vi "Teleop.vi"(10 "Match Info":T1={"Autonomous Elapsed Seconds"=0.0, "TeleOp Elapsed Seconds"=0.0, "Disabled Elapsed Seconds"=0.0, "Visited Autonomous"=FALSE, "Visited TeleOp"=FALSE, "Visited Disabled"=FALSE, "Autonomous Settings"={"Autonomous Style"=enum."Independent", "VI Refnum"=refnum}}, 11 "Call Context":T2) -> ()   [LabVIEW 2014]
doc: "This VI is called for each TeleOp packet received from the DS where the robot is not disabled. It is often used to read from the joysticks and update I/O or to update setpoints for timed control loops. It should complete and return within 20 milliseconds or it may miss DS packets."
uses:
  <vilib>/Rock Robotics/WPI/DriverStation/WPI_DriverStationDerivedRobotMode.ctl
  <vilib>/Rock Robotics/WPI/DriverStation/WPI_DriverStationMatch Info.ctl
  <vilib>/Rock Robotics/WPI/Solenoid/WPI_SolenoidValue.ctl
  <vilib>/Rock Robotics/WPI/RobotDrive/WPI_RobotDriveGetSetRefNum.vi
  <vilib>/Rock Robotics/WPI/Joystick/WPI_JoystickGetSetRefNum.vi
  Robot Global Data.vi
  <vilib>/Rock Robotics/WPI/Solenoid/WPI_SolenoidSetEnum.vi
  <vilib>/Rock Robotics/WPI/RobotDrive/WPI_RobotDriveArcadeDrive_Standard(NoSaturation).vi
panel:
  out "Pickup arm was down":bool
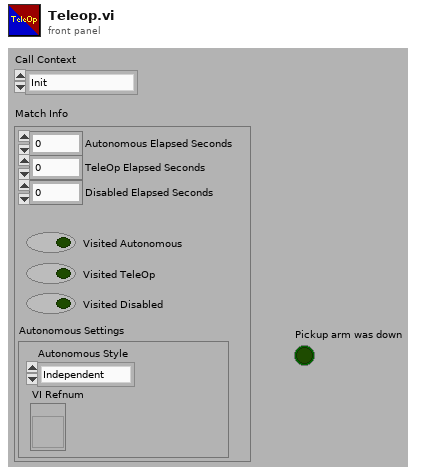
[diagram p1: front panel]
types:
  T1 = typedef "WPI_DriverStationMatch Info.ctl" = cluster{"Autonomous Elapsed Seconds":dbl, "TeleOp Elapsed Seconds":dbl, "Disabled Elapsed Seconds":dbl, "Visited Autonomous":bool, "Visited TeleOp":bool, "Visited Disabled":bool, "Autonomous Settings":cluster{"Autonomous Style":enum16{"Iterative", "Independent"}, "VI Refnum":refnum<vi>}}
  T2 = typedef "WPI_DriverStationDerivedRobotMode.ctl" = enum16{"Init", "Execute", "Stop"}
  T3 = typedef "WPI_SolenoidValue.ctl" = enum16{"Off", "On", "Forward", "Reverse"}
  T4 = typedef "WPI_JoystickDevRef.ctl" = cluster{"Device":T5}
  T5 = typedef "WPI_JoystickDeviceEnum.ctl" = enum16{"USB 0", "USB 1", "USB 2", "USB 3", "USB 4", "USB 5"}
  T6 = cluster{"Button 1":bool, "Button 2":bool, "Button 3":bool, "Button 4":bool, "Button 5":bool, "Button 6":bool, "Button 7":bool, "Button 8":bool, "Button 9":bool, "Button 10":bool, "Button 11":bool, "Button 12":bool}
  T7 = cluster{"axis 1 (x)":dbl, "axis 2 (y)":dbl, "axis 3 (throttle)":dbl, "axis 4":dbl, "axis 5":dbl, "axis 6":dbl}
  T8 = typedef "WPI_RobotDriveDevRef.ctl" = cluster{"DevStatus":errorcluster, "Motors[]":T9[], "Square Inputs":bool, "Max Output":dbl}
  T9 = typedef "WPI_MotorControlDeviceRef.ctl" = cluster{"DeviceStatus":errorcluster, "Type":enum16{"PWM", "CAN"}, "PWM":cluster{"Digital Module":T10, "PWM Channel":T11, "DeadBand":T12}, "CAN":cluster{"Device Number":u8, "Control Mode":T13, "Semaphore":T14, "Max Vout":dbl}, "Invert":bool, "TransformRef":T15, "InvTransformRef":T15}
  T10 = typedef "FPGA_TypedefDigitalModule.ctl" = enum16{"Digital Module 1", "Digital Module 2"}
  T11 = typedef "FPGA_DIOPWMChannel.ctl" = enum8{"PWM 1", "PWM 2", "PWM 3", "PWM 4", "PWM 5", "PWM 6", "PWM 7", "PWM 8", "PWM 9", "PWM 10", "Invalid"}
  T12 = typedef "WPI_PWMDeadband.ctl" = cluster{"Name":string, "maxPositivePwm":i32, "minPositivePwm":i32, "centerPwm":i32, "maxNegativePwm":i32, "minNegativePwm":i32, "angularRange":u16}
  T13 = typedef "WPI_CANJaguar_ControlMode.ctl" = enum8{"Percent VBus", "Current", "Speed", "Position", "Voltage"}
  T14 = typedef "Semaphore RefNum" = refnum<k1>
  T15 = typedef "WPI_PWMTransform_ConPane.ctl" = refnum<vi>
  T16 = typedef "WPI_SolenoidDevRef.ctl" = cluster{"DevStatus":errorcluster, "Solenoid Module":T17, "Forward Solenoid Channel":T18, "Reverse Solenoid Channel":T18}
  T17 = typedef "FPGA_TypedefSolenoidModule.ctl" = enum16{"Solenoid Module 1", "Solenoid Module 2"}
  T18 = typedef "WPI_SolenoidChannel.ctl" = enum8{"Solenoid 1", "Solenoid 2", "Solenoid 3", "Solenoid 4", "Solenoid 5", "Solenoid 6", "Solenoid 7", "Solenoid 8", "Invalid"}
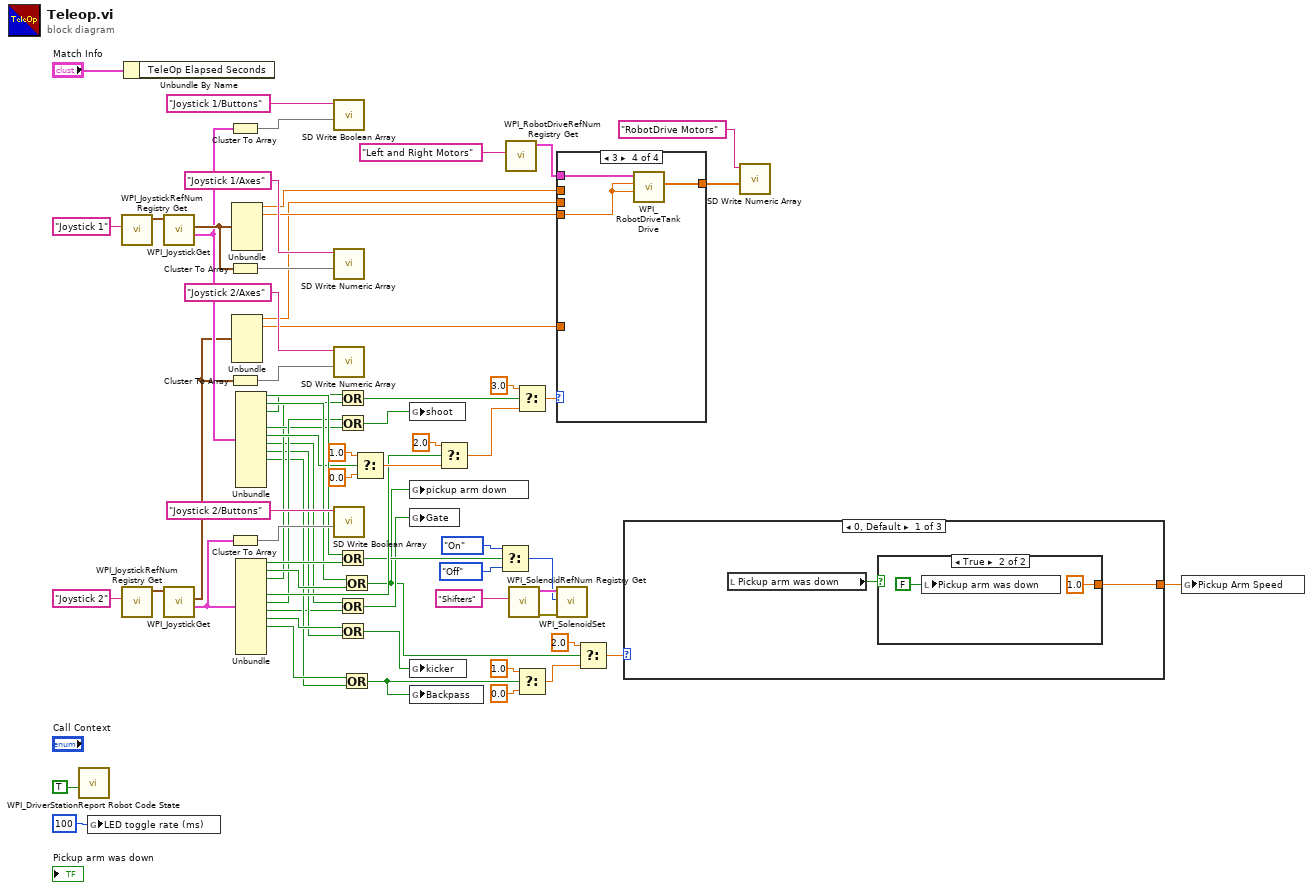
[diagram p0: block diagram]
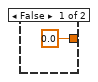
[diagram p2: hidden frame]
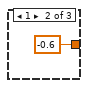
[diagram p3: hidden frame]
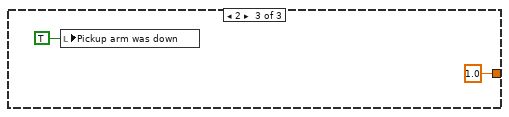
[diagram p4: hidden frame]
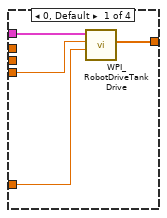
[diagram p5: hidden frame]
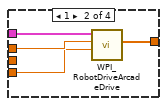
[diagram p6: hidden frame]
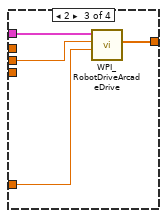
[diagram p7: hidden frame]
diagram:
  n1 = call <vilib>:"WPI_DriverStationReport Robot Code State.vi"("TeleOp"=TRUE ("Autonomous")) -> ()  [unwired: 10 in, 1 out]
  n2 = global write "Robot Global Data.vi" "LED toggle rate (ms)"(u32 100 ("LED ms toggle rate")) -> ()
  n3 = call <vilib>:"WPI_JoystickRefNum Registry Get.vi"("refnum name"="Joystick 1") -> ("JoystickDevRef"=w66:T4)  [unwired: 1 in, 9 out]
  n4 = call <vilib>:"WPI_JoystickRefNum Registry Get.vi"("refnum name"="Joystick 2") -> ("JoystickDevRef"=w58:T4)  [unwired: 1 in, 9 out]
  n5 = Unbundle By Name("Match Info") -> ()  [unwired: 1 out]
  n6 = call <vilib>:"WPI_JoystickGet.vi"("JoystickDevRef"=w66) -> ("Buttons"=w49:T6, "Axes"=w52:T7)  [unwired: 1 in, 4 out]
  n7 = call <vilib>:"WPI_JoystickGet.vi"("JoystickDevRef"=w58) -> ("Buttons"=w47:T6, "Axes"=w48:T7)  [unwired: 1 in, 4 out]
  n8 = Cluster To Array(cluster=w49) -> (array=w63:bool[])
  n9 = Cluster To Array(cluster=w52) -> (array=w61:dbl[])
  n10 = Cluster To Array(cluster=w48) -> (array=w55:dbl[])
  n11 = Cluster To Array(cluster=w47) -> (array=w57:bool[])
  n12 = Unbundle(w52) -> ("axis 1 (x)"=w51:dbl, "axis 2 (y)"=w50:dbl)  [unwired: 4 out]
  n13 = Unbundle(w48) -> ("axis 1 (x)"=w42:dbl, "axis 2 (y)"=w41:dbl)  [unwired: 4 out]
  n14 = Unbundle(w49) -> ("Button 1"=w32:bool, "Button 2"=w30:bool, "Button 3"=w17:bool, "Button 5"=w19:bool, "Button 6"=w21:bool, "Button 7"=w11:bool, "Button 8"=w7:bool, "Button 9"=w8:bool)  [unwired: 4 out]
  n15 = Unbundle(w47) -> ("Button 1"=w33:bool, "Button 2"=w29:bool, "Button 3"=w16:bool, "Button 5"=w22:bool, "Button 6"=w20:bool, "Button 7"=w6:bool, "Button 8"=w10:bool, "Button 9"=w9:bool)  [unwired: 4 out]
  n16 = call <vilib>:"SD Write Boolean Array.vi"("Boolean Array"=w63, "Name"="Joystick 1/Buttons") -> ()  [unwired: 8 in, 2 out]
  n17 = call <vilib>:"SD Write Numeric Array.vi"("Numeric Array"=w61, "Name"="Joystick 1/Axes") -> ()  [unwired: 8 in, 2 out]
  n18 = call <vilib>:"SD Write Numeric Array.vi"("Numeric Array"=w55, "Name"="Joystick 2/Axes") -> ()  [unwired: 8 in, 2 out]
  n19 = call <vilib>:"SD Write Boolean Array.vi"("Boolean Array"=w57, "Name"="Joystick 2/Buttons") -> ()  [unwired: 8 in, 2 out]
  n20 = Or(x=w17, y=w16) -> (x .or. y?=w15:bool)
  n21 = Or(x=w20, y=w19) -> (x .or. y?=w2:bool)
  n22 = Or(x=w32, y=w33) -> (x .or. y?=w18:bool)
  n23 = Or(x=w11, y=w6) -> (x .or. y?=w5:bool)
  n24 = Or(x=w10, y=w7) -> (x .or. y?=w4:bool)
  n25 = Or(x=w30, y=w29) -> (x .or. y?=w1:bool)
  n26 = Or(x=w9, y=w8) -> (x .or. y?=w3:bool)
  n27 = Select(t=1.0, s=w21, f=0.0) -> (s? t:f=w46:dbl)
  n28 = global write "Robot Global Data.vi" "shoot"(w2) -> ()
  n29 = global write "Robot Global Data.vi" "pickup arm down"(w1) -> ()
  n30 = global write "Robot Global Data.vi" "Gate"(w5) -> ()
  n31 = global write "Robot Global Data.vi" "kicker"(w4) -> ()
  n32 = global write "Robot Global Data.vi" "Backpass"(w3) -> ()
  n33 = Select(t=2.0, s=w22, f=w46) -> (s? t:f=w13:dbl)
  n34 = Select(t=WPI_SolenoidValue."On" ("Value"), s=w18, f=WPI_SolenoidValue."Off" ("Value")) -> (s? t:f=w34:T3)
  n35 = call <vilib>:"WPI_RobotDriveRefNum Registry Get.vi"("refnum name"="Left and Right Motors") -> ("RobotDriveDevRef"=w40:T8)  [unwired: 1 in, 9 out]
  n36 = call <vilib>:"WPI_SolenoidRefNum Registry Get.vi"("refnum name"="Shifters") -> ("error out"=w38:errorcluster, "SolenoidDevRef"=w37:T16)  [unwired: 9 in]
  n37 = Select(t=3.0, s=w15, f=w13) -> (s? t:f=w12:dbl)
  n38 = Select(t=1.0, s=w3, f=0.0) -> (s? t:f=w25:dbl)
  n39 = case shown="3" w12 {
    tunnel: w51 -> [_ w76 _ _]
    tunnel: w50 -> [w73 w75 _ w82]
    tunnel: w42 -> [_ _ w79 _]
    tunnel: w41 -> [w72 _ w78 _]
    tunnel: w40 -> [w71 w77 w81 w84]
    tunnel: [w70 w74 w80 w83] -> w39
    frame 0, Default {
      n40 = call <vilib>:"WPI_RobotDriveTankDrive.vi"("Right axis value"=w72, "Left axis value"=w73, "RobotDriveDevRef"=w71) -> ("Motor Values"=w70:dbl[])  [unwired: 6 in, 2 out]
    }
    frame 1 {
      n41 = call-poly <vilib>:"WPI_RobotDriveArcadeDrive.vi"("Y axis value"=w75, "X axis value"=w76, "RobotDriveDevRef"=w77) -> ("Motor Values"=w74:dbl[])  [unwired: 6 in, 2 out]
    }
    frame 2 {
      n42 = call-poly <vilib>:"WPI_RobotDriveArcadeDrive.vi"("Y axis value"=w78, "X axis value"=w79, "RobotDriveDevRef"=w81) -> ("Motor Values"=w80:dbl[])  [unwired: 6 in, 2 out]
    }
    frame 3 {
      n43 = call <vilib>:"WPI_RobotDriveTankDrive.vi"("Right axis value"=w82, "Left axis value"=w82, "RobotDriveDevRef"=w84) -> ("Motor Values"=w83:dbl[])  [unwired: 6 in, 2 out]
    }
  }
  n44 = call-poly <vilib>:"WPI_SolenoidSet.vi"("error in (no error)"=w38, "Value"=w34, "SolenoidDevRef"=w37) -> ()  [unwired: 7 in, 2 out]
  n45 = Select(t=2.0, s=w1, f=w25) -> (s? t:f=w24:dbl)
  n46 = case shown="0, Default" w24 {
    tunnel: [w86 -0.6 ("f") 1.0 ("f")] -> w23
    frame 0, Default {
      n47 = local read "Pickup arm was down"() -> (w85:bool)
      n48 = case shown="True" w85 {
        tunnel: [0.0 ("f") 1.0 ("f")] -> w86
        frame False {
        }
        frame True {
          n49 = local write "Pickup arm was down"(FALSE ("Pickup arm was down")) -> ()
        }
      }
    }
    frame 1 {
    }
    frame 2 {
      n50 = local write "Pickup arm was down"(TRUE ("Pickup arm was down")) -> ()
    }
  }
  n51 = call <vilib>:"SD Write Numeric Array.vi"("Numeric Array"=w39, "Name"="RobotDrive Motors") -> ()  [unwired: 8 in, 2 out]
  n52 = global write "Robot Global Data.vi" "Pickup Arm Speed"(w23) -> ()
